vi "RT_P3.vi"() -> ()   [LabVIEW 2014]
uses:
  <vilib>/Utility/RT CPU Load.ctl
  <vilib>/Platform/TimedLoop/XDataNode/timing_clust.ctl
  <vilib>/Platform/TimedLoop/XDataNode/nitl_modes.ctl
  <vilib>/Platform/TimedLoop/XDataNode/wakeup.ctl
  <vilib>/RioEmbeddedCAN/RioEmbeddedCAN.llb/CANFilterMode.ctl
  <vilib>/RioEmbeddedCAN/RioEmbeddedCAN.llb/CANFilterSetting.ctl
  <vilib>/FPGAPlugInAG/sbRIO-9636/niLvFpga_Open_sbRIO-9636.vi
  <vilib>/FPGAPlugInAG/sbRIO-9636/niLvFpga_Close_sbRIO-9636.vi
  <vilib>/Instr/_visa.llb/VISA Configure Serial Port (Instr).vi
  <vilib>/rvi/interface/common/dynamic/niFpgaDynamicAddResources.vi
  <vilib>/FPGAPlugInAG/Dynamic/niLvFpga_Reset_Dynamic.vi
  <vilib>/FPGAPlugInAG/Dynamic/niLvFpga_Run_Dynamic.vi
  <vilib>/Utility/error.llb/Error Cluster From Error Code.vi
  <vilib>/rvi/errors/niLvFpgaAdjustHostInterfaceError.vi
  <vilib>/FPGAPlugInAG/Dynamic/niLvFpga_Close_Dynamic.vi
  <vilib>/Platform/TimedLoop/XDataNode/XDataNode.xnode
  Z:/cloud/LabView/roger-i2c/Host API/Controls/FPGA I2C_FPGA Ref.ctl
  <vilib>/rvi/interface/nirviOpenFPGA/nirviOpenFPGA.xnode
  FPGA bitfiles/telemetriap3_FPGATarget_fpgaprova_w0avayymtNg.lvbitx
  fpga_p3.vi
  <vilib>/rvi/interface/nirviCloseFPGA/nirviCloseFPGA.xnode
  <vilib>/rvi/interface/nirviMethod/nirviMethod.xnode
  <vilib>/rvi/interface/nirviReadWriteControl/nirviReadWriteControl.xnode
  <vilib>/Platform/TimedLoop/XDataNode/XDNodeRunTimeDep.lvlib
  <vilib>/NI_Real-Time Target Support.lvlib
  <vilib>/FPGAPlugInAG/Dynamic/niLvFpga_ReadFifo_Dynamic.vi
  <vilib>/rvi/errors/niLvFpgaMergeErrorWithErrorCode.vi
  <vilib>/FPGAPlugInAG/Dynamic/niLvFpga_StartFifo_Dynamic.vi
  NiFpgaLv.dll
  <vilib>/rvi/interface/Simulation/niFpgaSimulationCallBeginRW.vi
panel:
  out "a-z":dbl
  out "a-y":dbl
  out "a-x":dbl
  out "CPU loads":T1[](array[typedef]) {"ISR (%)" format="%#.2f"; "Idle (%)" format="%#.2f"; "Background (%)" format="%#.2f"; "Normal (%)" format="%#.2f"; "Above Normal (%)" format="%#.2f"; "High (%)" format="%#.2g"; "Timed Structures (%)" format="%#.2g"; "Time Critical (%)" format="%#.2g"; "Total (%)" format="%#.2g"}
  out "g-z":dbl
  out "g-y":dbl
  out "g-x":dbl
  out "Error rs-232 display":errorcluster
  in  "Buzzer":bool
  in  "STOP LIGHT":bool
  out "Brake Sensor \nFront":sgl
  out "error out save file":errorcluster
  out "Brake Sensor \nRear":sgl
  out "Steering anlge":sgl
  out "overflow?":bool
  in  "stop":bool
  out "=< 10?":bool
  out "Loop Time":u32
  out "Fifo Overflow?":bool
  out "Elements Remaining after":u32
  out "F-L":sgl
  out "R-R":sgl
  out "F-R":sgl
  out "R-L":sgl
  out "Elements Remaining before":u32
  out "error out fpga":errorcluster
  out "Drive Speed":sgl
  out "Fuel Used":sgl
  out "Gear":u16
  out "Oil Temp":sgl
  out "Oil Pressure":sgl
  out "Battery Voltage":sgl
  out "Engine Temp":sgl
  out "Throttle":sgl
  out "Lambda":sgl
  out "Air Temp":sgl
  out "Map (bar)":sgl
  out "Rpm":u16
  out "error out can":errorcluster
  # "CAN MOTEC"
  # "FPGA"
  # "Telemetria delle telemetria"
  # "I2C\nI2C\nI2C Sistema inerziale"
  # "Indirizzo 2"
  # "Indirizzo 3"
  # "Indirizzo 4"
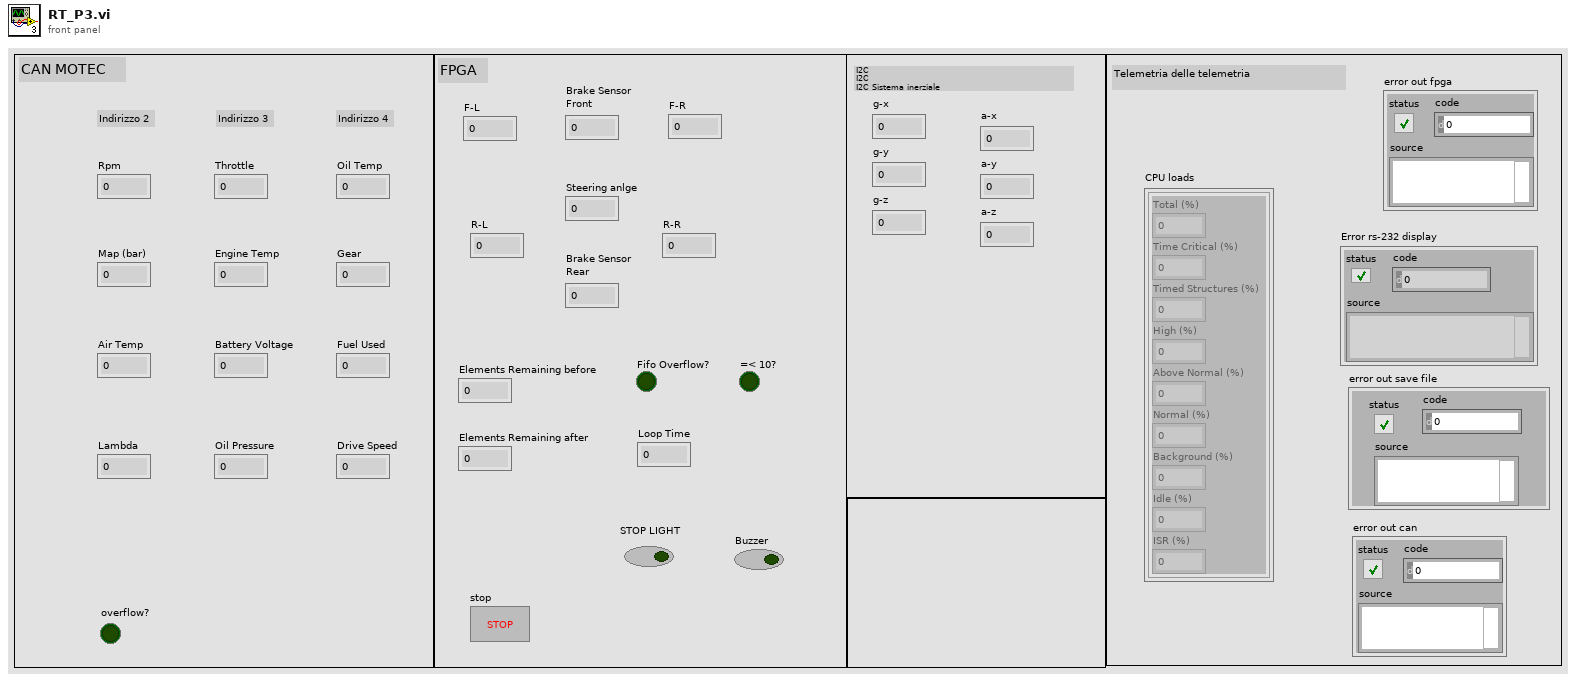
[diagram p1: front panel]
types:
  T1 = typedef "NI_Real-Time Target Support.lvlib/RT CPU Load.ctl" = cluster{"Total (%)":dbl, "Time Critical (%)":dbl, "Timed Structures (%)":dbl, "High (%)":dbl, "Above Normal (%)":dbl, "Normal (%)":dbl, "Background (%)":dbl, "Idle (%)":dbl, "ISR (%)":dbl}
  T2 = typedef "XDNodeRunTimeDep.lvlib/timing_clust.ctl" = cluster{"Expected End [f-1]":u64, "Actual End [f-1]":u64, "Finished Late? [f-1]":bool, "Expected End [i-1]":u64, "Actual End [i-1]":u64, "Finished Late? [i-1]":bool, "Expected Start [i]":u64, "Actual Start [i]":u64, "Expected Start [f]":u64, "Actual Start [f]":u64, "Source Name":string, "Structure Name":string, "Period":i64, "Deadline":i64, "Offset":i64, "Start":i64, "Priority":i32, "Timeout":i32, "Mode":T3, "Wakeup Reason":T4, "Error":errorcluster, "Source Type":string, "Secondary Source Type":string, "Global End Time":u64, "Global Start Time":u64, "Frame Duration":u64, "Iteration Duration":u64, "Assigned CPU":i32, "I/O Scan Engine Mode":u32}
  T3 = typedef "XDNodeRunTimeDep.lvlib/nitl_modes.ctl" = enum32{"No Change", "Process missed periods, maintain original phase", "Discard missed periods, maintain original phase", "Process missed periods, ignore original phase", "Discard missed periods, ignore original phase"}
  T4 = typedef "XDNodeRunTimeDep.lvlib/wakeup.ctl" = enum32{"Normal", "Aborted", "Asynchronous wakeup", "Timing source error", "Timed loop error", "Timeout"}
  T5 = typedef "CANFilterSetting.ctl" = cluster{"identifier":u32, "identifier mask":u32, "extended?":bool, "RTR?":bool, "RTR mask?":bool}
  T6 = typedef "CANFilterMode.ctl" = enum16{"Disabled", "32-bit", "16-bit", "8-bit"}
  T7 = typedef "CANFrameControl.ctl" = cluster{"identifier":u32, "extended?":bool, "type":u8, "payload":u8[]}
  T8 = enum16{"open", "open or create", "create or replace", "create", "open (read-only)"}
  T9 = typedef "FPGA I2C_FPGA Ref.ctl" = refnum<k20>
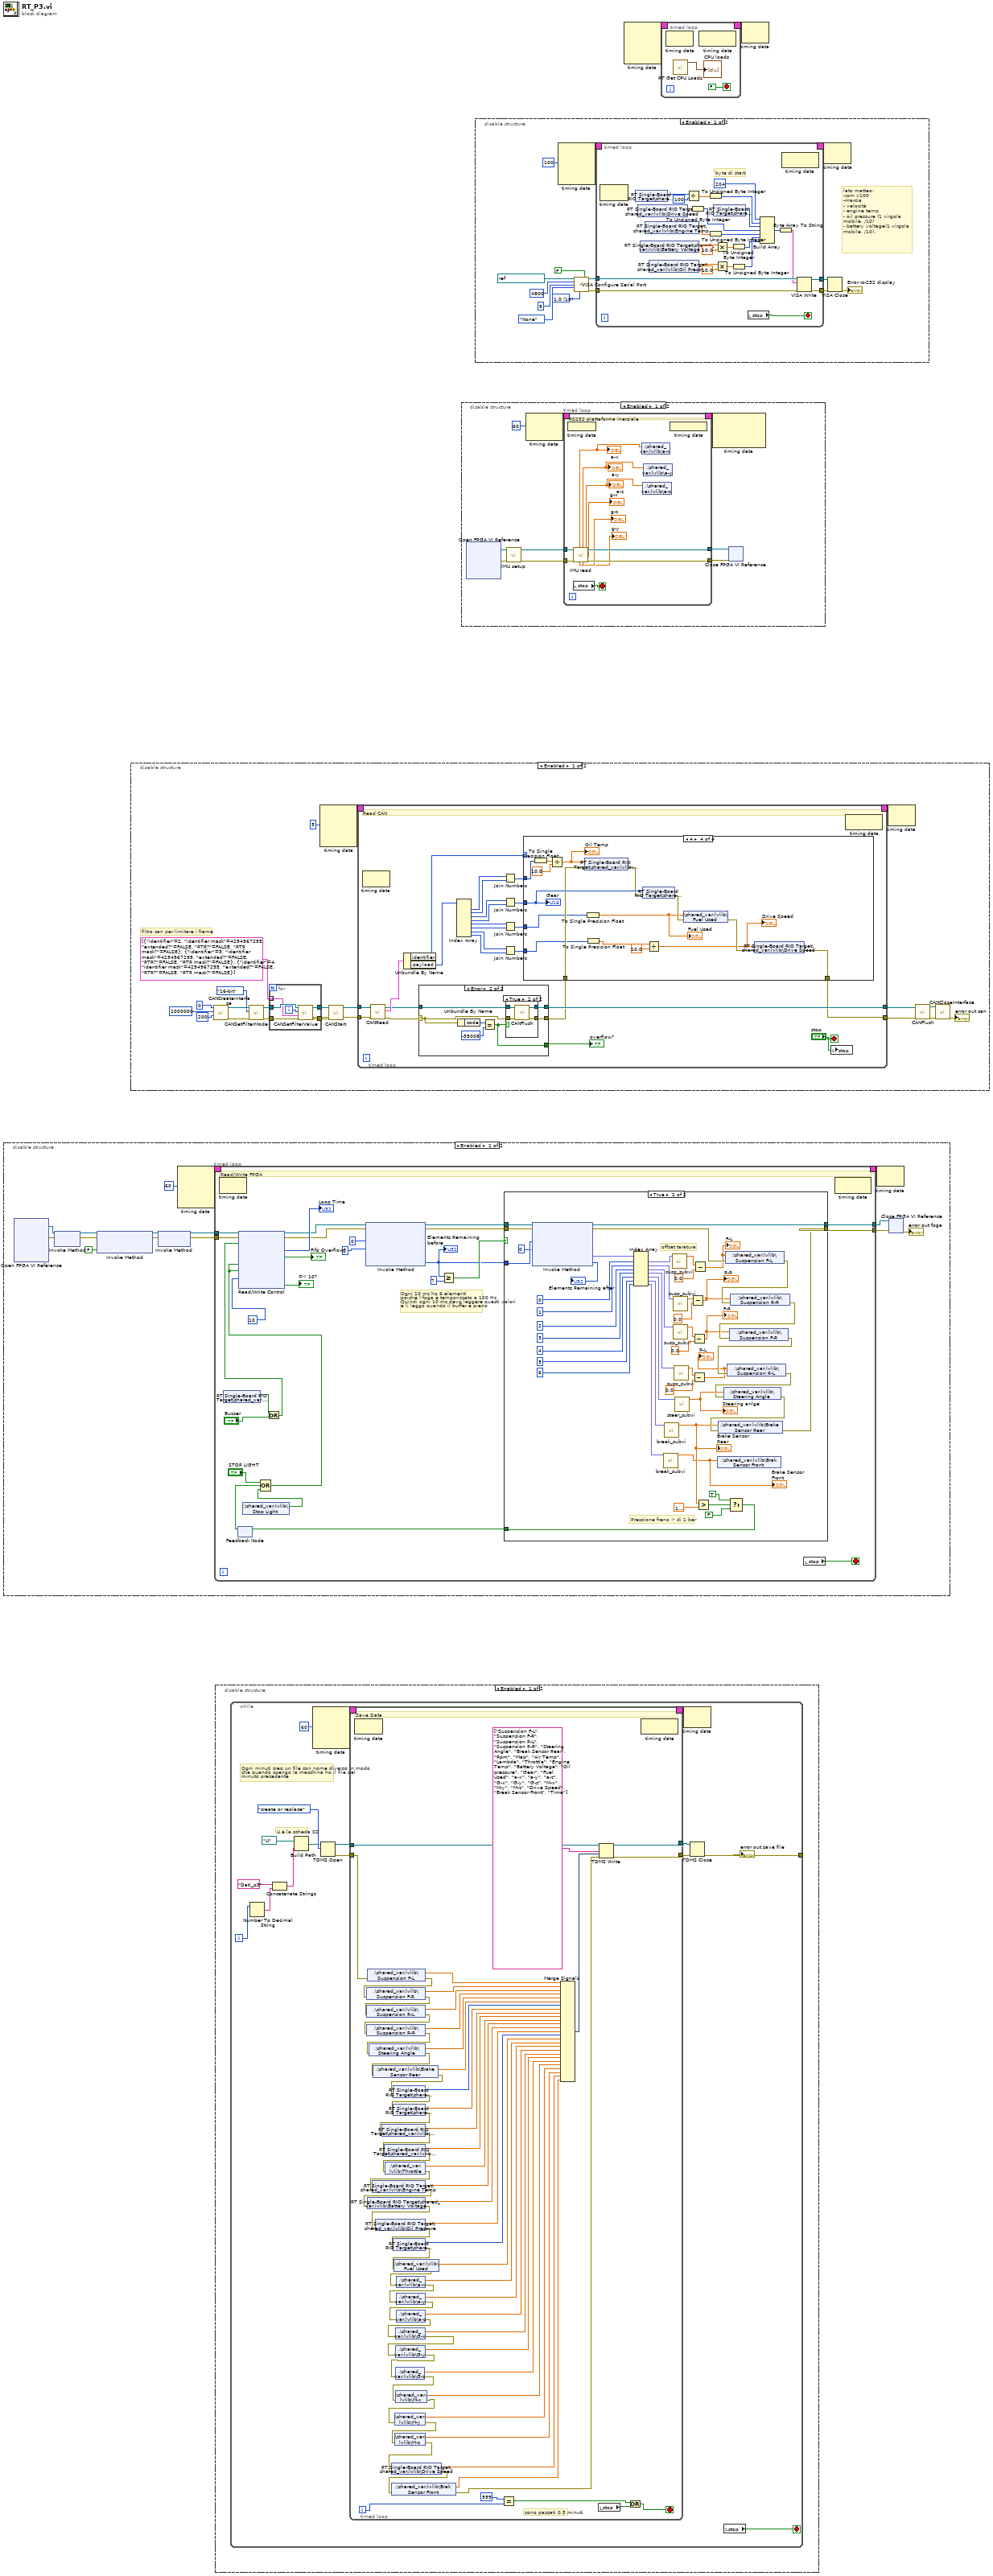
[diagram p0: block diagram]
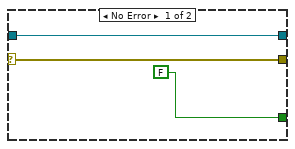
[diagram p4: hidden frame]
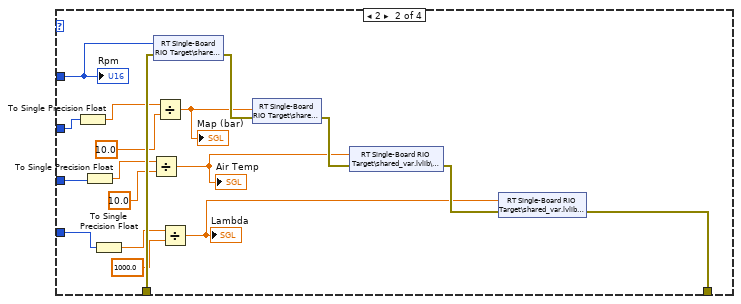
[diagram p7: hidden frame]
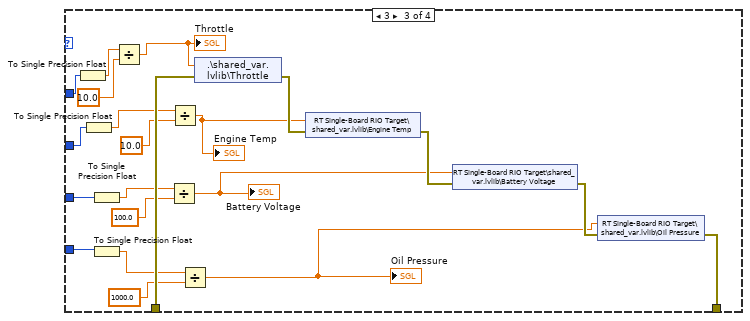
[diagram p8: hidden frame]
diagram:
  n1 = disable-structure shown="Enabled" {
    frame Enabled {
      n2 = xnode "Open FPGA VI Reference"() -> ("FPGA VI Reference Out"=w15:refnum<k20>, "error out"=w14:errorcluster)  [unwired: 2 in]
      n3 = xnode "Invoke Method"("FPGA VI Reference In"=w15, "error in"=w14) -> ("FPGA VI Reference Out"=w12:refnum<k20>, "error out"=w11:errorcluster)
      n4 = xnode "Invoke Method"("FPGA VI Reference In"=w12, "error in"=w11, "Wait Until Done (F)"=FALSE) -> ("FPGA VI Reference Out"=w7:refnum<k20>, "error out"=w6:errorcluster)
      n5 = xnode "Invoke Method"("FPGA VI Reference In"=w7, "error in"=w6) -> ("FPGA VI Reference Out"=w5:refnum<k20>, "error out"=w4:errorcluster)
      n6 = node-c288(i64 60 ("Period")) -> (w17:T2)  [unwired: 3 in]
      n7 = timed-loop {
        tunnel: [w33] -> w9
        tunnel: [w32] -> w8
        tunnel: w5 -> [w31]
        tunnel: w4 -> [w30]
        timing: w17 -> [_]
        timing-out: [_] -> w16
        stop <- w27 stop-if-true
        # "Ogni 10 ms ho 6 elementi\npoichè l'fpga è temporizzato a 100 Hz\nQuindi ogni 10 ms devo leggere questi valori\ne li leggo quando il buffer è pieno"
        # "Read/Write FPGA"
        n8 = node-c288() -> ()  [unwired: 1 in, 1 out]
        n9 = shared-variable "RT Single-Board RIO Target\\shared_var.lvlib\\Buzzer"() -> (w23:bool)  [unwired: 1 in, 1 out]
        n10 = feedback #1() -> (w19:bool)  [unwired: 1 in]
        n11 = shared-variable ".\\shared_var.lvlib\\Stop Light"() -> (w18:bool)  [unwired: 1 in, 1 out]
        n12 = Compound Arithmetic op=OR("STOP LIGHT", w19, w18) -> (w21:bool)
        n13 = Or(x=w23, y="Buzzer") -> (x .or. y?=w22:bool)
        n14 = xnode "Read/Write Control"("FPGA VI Reference In"=w31, "error in"=w30, "Buzzer"=w22, "FPGA LED"=w21, "Stop Light"=w21, "Count(uSec)"=u32 10 ("Count(mSec)")) -> ("FPGA VI Reference Out"=w29:refnum<k20>, "error out"=w34:errorcluster, "Loop Time"=→"Loop Time":u32, "Fifo Overflow?"=→"Fifo Overflow?":bool, "=< Lopp time?"=→"=< 10?":bool)
        n15 = xnode "Invoke Method"("FPGA VI Reference In"=w29, "error in"=w34, "Number of Elements"=u32 0, "Timeout (ms)"=0) -> ("FPGA VI Reference Out"=w40:refnum<k20>, "error out"=w39:errorcluster, "Elements Remaining"=w35:u32)  [unwired: 1 out]
        "Elements Remaining before" <- w35
        n16 = Greater Or Equal?(x=w35, y=u32 7) -> (x >= y?=w37:bool)
        n17 = case shown="True" w37 {
          tunnel: w40 -> [w47 w95]
          tunnel: w39 -> [w46 w94]
          tunnel: [w47 w93] -> w33
          tunnel: [w46 w83] -> w32
          tunnel: w35 -> [_ w92]
          tunnel: [_ w88] -> w28
          frame False {
          }
          frame True {
            # "offset taratura"
            # "Pressione freno > di 1 bar"
            n18 = xnode "Invoke Method"("FPGA VI Reference In"=w95, "error in"=w94, "Number of Elements"=w92, "Timeout (ms)"=0) -> ("FPGA VI Reference Out"=w93:refnum<k20>, "error out"=w85:errorcluster, "Data"=w82:fxp<+,32,3>[], "Elements Remaining"=→"Elements Remaining after":u32)
            n19 = Index Array(array=w82, index #1=0 ("index"), index #2=1 ("index"), index #3=2 ("index"), index #4=3 ("index"), index #5=4 ("index"), index #6=5 ("index"), index #7=6 ("index")) -> (element #1=w73:fxp<+,32,3>, element #2=w72:fxp<+,32,3>, element #3=w71:fxp<+,32,3>, element #4=w70:fxp<+,32,3>, element #5=w69:fxp<+,32,3>, element #6=w67:fxp<+,32,3>, element #7=w49:fxp<+,32,3>)
            n20 = call "break_subvi.vi"("Numeric in"=w49) -> ("Numeric out"=w48:sgl)  [unwired: 10 in]
            "Brake Sensor \nFront" <- w48
            n21 = call "break_subvi.vi"("Numeric in"=w67) -> ("Numeric out"=w50:sgl)  [unwired: 10 in]
            "Brake Sensor \nRear" <- w50
            n22 = call "susp_subvi.vi"("Numeric in"=w73) -> ("Numeric out"=w62:sgl)  [unwired: 10 in]
            n23 = call "susp_subvi.vi"("Numeric in"=w72) -> ("Numeric out"=w55:sgl)  [unwired: 10 in]
            n24 = call "susp_subvi.vi"("Numeric in"=w71) -> ("Numeric out"=w59:sgl)  [unwired: 10 in]
            n25 = call "susp_subvi.vi"("Numeric in"=w70) -> ("Numeric out"=w53:sgl)  [unwired: 10 in]
            n26 = call "steer_subvi.vi"("Numeric in"=w69) -> ("Numeric out"=w68:sgl)  [unwired: 10 in]
            "Steering anlge" <- w68
            n27 = Subtract(x=w55, y=sgl 0.0 ("Off R-R")) -> (x-y=w56:sgl)
            "R-R" <- w56
            n28 = Subtract(x=w59, y=sgl 0.0 ("Off F-R")) -> (x-y=w58:sgl)
            "F-R" <- w58
            n29 = Subtract(x=w53, y=sgl 0.0 ("Off R-L")) -> (x-y=w52:sgl)
            "R-L" <- w52
            n30 = Subtract(x=w62, y=sgl 0.0 ("Off F-L")) -> (x-y=w61:sgl)
            "F-L" <- w61
            n31 = Greater?(x=w50, y=sgl 1.7) -> (0:w89:bool)
            n32 = shared-variable ".\\shared_var.lvlib\\Brak Sensor Front"(w48) -> ()  [unwired: 1 in, 1 out]
            n33 = shared-variable ".\\shared_var.lvlib\\Suspension F-L"(w61, error in=w85) -> (error out=w66:errorcluster)
            n34 = Select(t=TRUE, s=w89, f=FALSE) -> (s? t:f=w88:bool)
            n35 = shared-variable ".\\shared_var.lvlib\\Suspension R-R"(w56, error in=w66) -> (error out=w65:errorcluster)
            n36 = shared-variable ".\\shared_var.lvlib\\Suspension F-R"(w58, error in=w65) -> (error out=w63:errorcluster)
            n37 = shared-variable ".\\shared_var.lvlib\\Suspension R-L"(w52, error in=w63) -> (error out=w64:errorcluster)
            n38 = shared-variable ".\\shared_var.lvlib\\Steering Angle"(w68, error in=w64) -> (error out=w84:errorcluster)
            n39 = shared-variable ".\\shared_var.lvlib\\Brake Sensor Rear"(w50, error in=w84) -> (error out=w83:errorcluster)
          }
        }
        n40 = feedback-in #1(w28) -> ()
        n41 = local read "stop"() -> (w27:bool)
        n42 = node-c288() -> ()  [unwired: 1 in, 1 out]
      }
      n43 = node-c288(w16) -> ()  [unwired: 1 out]
      n44 = xnode "Close FPGA VI Reference"("FPGA VI Reference In"=w9, "error in"=w8) -> ("error out"=→"error out fpga":errorcluster)
    }
    frame Disabled {
    }
  }
  n45 = disable-structure shown="Enabled" {
    frame Enabled {
      # "filtro can per limitare i frame"
      n46 = call <vilib>:"CANCreateInterface.vi"("receive queue size (5)"=u32 200, "baud rate (125000 bps)"=u32 1000000, "interface index"=u32 0) -> ("error out"=w115:errorcluster, "interface object out"=w116:refnum<k20>)  [unwired: 7 in]
      n47 = call <vilib>:"CANSetFilterMode.vi"("error in (no error)"=w115, "filter mode (32-bit)"=CANFilterMode."16-bit", "interface object in"=w116) -> ("error out"=w117:errorcluster, "interface object out"=w118:refnum<k20>)  [unwired: 7 in]
      n48 = for {
        tunnel: T5[] [{"identifier"=2, "identifier mask"=4294967295, "extended?"=FALSE, "RTR?"=FALSE, "RTR mask?"=FALSE}, {"identifier"=3, "identifier mask"=4294967295, "extended?"=FALSE, "RTR?"=FALSE, "RTR mask?"=FALSE}, {"identifier"=4, "identifier mask"=4294967295, "extended?"=FALSE, "RTR?"=FALSE, "RTR mask?"=FALSE}] ("Array") -> [w225] mode=indexing
        tunnel: w118 -> [w228]
        tunnel: [w227] -> w113
        tunnel: w117 -> [w223]
        tunnel: [w226] -> w112
        i -> [w224]
        n49 = call <vilib>:"CANSetFilterValue.vi"("error in (no error)"=w223, "filter frame"=w225, "filter index (0)"=w224, "interface object in"=w228) -> ("error out"=w226:errorcluster, "interface object out"=w227:refnum<k20>)  [unwired: 6 in]
      }
      n50 = node-c288(i64 5 ("Period")) -> (w120:T2)  [unwired: 3 in]
      n51 = call <vilib>:"CANStart.vi"("error in (no error)"=w112, "interface object in"=w113) -> ("error out"=w110:errorcluster, "interface object out"=w111:refnum<k20>)  [unwired: 8 in]
      n52 = timed-loop {
        tunnel: w111 -> [w143]
        tunnel: w110 -> [w144]
        tunnel: [w126] -> w104
        timing: w120 -> [_]
        timing-out: [_] -> w119
        tunnel: [w127] -> w102
        stop <- "stop" stop-if-true
        # "Read CAN"
        n53 = node-c288() -> ()  [unwired: 1 in, 1 out]
        n54 = call <vilib>:"CANRead.vi"("error in (no error)"=w144, "interface object in"=w143) -> ("error out"=w125:errorcluster, "CAN frame"=w142:T7, "interface object out"=w121:refnum<k20>)  [unwired: 6 in, 1 out]
        n55 = Unbundle By Name(w142) -> ("identifier"=w132:u32, "payload"=w133:u8[])
        n56 = case shown="Error" w125 {
          selector: w125 -> [w147 w150]
          tunnel: [w147 w151] -> w124
          tunnel: w121 -> [w146 w148]
          tunnel: [w146 w152] -> w127
          tunnel: [FALSE w149] -> w122
          frame No Error {
          }
          frame Error {
            n57 = Unbundle By Name(w150) -> ("code"=w154:i32)
            n58 = Equal?(x=w154, y=-35008) -> (x = y?=w149:bool)
            n59 = case shown="True" w149 {
              tunnel: w150 -> [w156 w158]
              tunnel: w148 -> [w155 w160]
              tunnel: [w155 w159] -> w152
              tunnel: [w156 w157] -> w151
              frame False {
              }
              frame True {
                n60 = call <vilib>:"CANFlush.vi"("error in (no error)"=w158, "interface object in"=w160) -> ("error out"=w157:errorcluster, "interface object out"=w159:refnum<k20>)  [unwired: 8 in]
              }
            }
          }
        }
        "overflow?" <- w122
        n61 = Index Array(array=w133) -> (element #1=w141:u8, element #2=w140:u8, element #3=w139:u8, element #4=w138:u8, element #5=w137:u8, element #6=w136:u8, element #7=w135:u8, element #8=w134:u8)  [unwired: 8 in]
        n62 = Join Numbers(hi=w141, lo=w140) -> ((hi.lo)=w131:u16)
        n63 = Join Numbers(hi=w139, lo=w138) -> ((hi.lo)=w130:u16)
        n64 = Join Numbers(hi=w137, lo=w136) -> ((hi.lo)=w129:u16)
        n65 = Join Numbers(hi=w135, lo=w134) -> ((hi.lo)=w128:u16)
        n66 = case shown="4" w132 {
          tunnel: w131 -> [_ w181 w196 w213]
          tunnel: w130 -> [_ w166 w190 w218]
          tunnel: w129 -> [_ w175 w195 w209]
          tunnel: w128 -> [_ w173 w185 w210]
          tunnel: w124 -> [w163 w180 w202 w217]
          tunnel: [w163 w176 w198 w207] -> w126
          frame 0, Default {
          }
          frame 2 {
            n67 = To Single Precision Float(number=w166) -> (single precision float=w165:sgl)
            n68 = To Single Precision Float(number=w175) -> (single precision float=w168:sgl)
            n69 = To Single Precision Float(number=w173) -> (single precision float=w170:sgl)
            n70 = Divide(x=w168, y=sgl 10.0 ("x")) -> (x/y=w174:sgl)
            "Air Temp" <- w174
            n71 = shared-variable "RT Single-Board RIO Target\\shared_var.lvlib\\Rpm"(w181, error in=w180) -> (error out=w179:errorcluster)
            n72 = Divide(x=w165, y=sgl 10.0 ("x")) -> (x/y=w164:sgl)
            "Map (bar)" <- w164
            n73 = Divide(x=w170, y=sgl 1000.0 ("x")) -> (x/y=w172:sgl)
            "Lambda" <- w172
            n74 = shared-variable "RT Single-Board RIO Target\\shared_var.lvlib\\Map"(w164, error in=w179) -> (error out=w178:errorcluster)
            n75 = shared-variable "RT Single-Board RIO Target\\shared_var.lvlib\\Air Temp"(w174, error in=w178) -> (error out=w177:errorcluster)
            n76 = shared-variable "RT Single-Board RIO Target\\shared_var.lvlib\\Lambda"(w172, error in=w177) -> (error out=w176:errorcluster)
            "Rpm" <- w181
          }
          frame 3 {
            n77 = To Single Precision Float(number=w196) -> (single precision float=w192:sgl)
            n78 = To Single Precision Float(number=w190) -> (single precision float=w187:sgl)
            n79 = To Single Precision Float(number=w195) -> (single precision float=w191:sgl)
            n80 = To Single Precision Float(number=w185) -> (single precision float=w184:sgl)
            n81 = Divide(x=w192, y=sgl 10.0 ("x")) -> (x/y=w197:sgl)
            "Throttle" <- w197
            n82 = Divide(x=w191, y=sgl 100.0) -> (x/y=w194:sgl)
            "Battery Voltage" <- w194
            n83 = Divide(x=w187, y=sgl 10.0 ("x")) -> (x/y=w189:sgl)
            "Engine Temp" <- w189
            n84 = Divide(x=w184, y=1000.0 ("x")) -> (x/y=w183:dbl)
            "Oil Pressure" <- w183
            n85 = shared-variable ".\\shared_var.lvlib\\Throttle"(w197, error in=w202) -> (error out=w201:errorcluster)
            n86 = shared-variable "RT Single-Board RIO Target\\shared_var.lvlib\\Engine Temp"(w189, error in=w201) -> (error out=w200:errorcluster)
            n87 = shared-variable "RT Single-Board RIO Target\\shared_var.lvlib\\Battery Voltage"(w194, error in=w200) -> (error out=w199:errorcluster)
            n88 = shared-variable "RT Single-Board RIO Target\\shared_var.lvlib\\Oil Pressure"(w183, error in=w199) -> (error out=w198:errorcluster)
          }
          frame 4 {
            n89 = To Single Precision Float(number=w213) -> (single precision float=w212:sgl)
            n90 = Divide(x=w212, y=sgl 10.0) -> (x/y=w214:sgl)
            "Oil Temp" <- w214
            n91 = shared-variable "RT Single-Board RIO Target\\shared_var.lvlib\\Oil Temp"(w214, error in=w217) -> (error out=w216:errorcluster)
            n92 = To Single Precision Float(number=w209) -> (single precision float=w206:sgl)
            "Fuel Used" <- w206
            n93 = To Single Precision Float(number=w210) -> (single precision float=w205:sgl)
            n94 = shared-variable "RT Single-Board RIO Target\\shared_var.lvlib\\Gear"(w218, error in=w216) -> (error out=w215:errorcluster)
            n95 = Divide(x=w205, y=sgl 10.0) -> (x/y=w204:sgl)
            "Drive Speed" <- w204
            n96 = shared-variable ".\\shared_var.lvlib\\Fuel Used"(w206, error in=w215) -> (error out=w208:errorcluster)
            n97 = shared-variable "RT Single-Board RIO Target\\shared_var.lvlib\\Drive Speed"(w204, error in=w208) -> (error out=w207:errorcluster)
            "Gear" <- w218
          }
        }
        n98 = local write "stop"("stop") -> ()
        n99 = node-c288() -> ()  [unwired: 1 in, 1 out]
      }
      n100 = node-c288(w119) -> ()  [unwired: 1 out]
      n101 = call <vilib>:"CANFlush.vi"("error in (no error)"=w104, "interface object in"=w102) -> ("error out"=w103:errorcluster, "interface object out"=w105:refnum<k20>)  [unwired: 8 in]
      n102 = call <vilib>:"CANCloseInterface.vi"("error in (no error)"=w103, "interface object in"=w105) -> ("error out"=→"error out can":errorcluster)  [unwired: 9 in]
    }
    frame Disabled {
    }
  }
  n103 = disable-structure shown="Enabled" {
    frame Enabled {
      n104 = while {
        tunnel: [w235] -> w229
        i -> [w234]
        stop <- w241 stop-if-true
        # "Ogni minuti creo un file con nome diverso in modo\nche quando spengo la macchina ho il file del \nminuto precedente"
        # "U è la scheda SD"
        n105 = Number To Decimal String(number=w234) -> (decimal integer string=w238:string)  [unwired: 1 in]
        n106 = Concatenate Strings("Dati_p3" ("name or relative path"), w238) -> (w239:string)
        n107 = Build Path(base path=path "U:/", name or relative path=w239) -> (appended path=w233:path)
        n108 = node-c288(i64 60 ("Period")) -> (w232:T2)  [unwired: 3 in]
        n109 = TDMS Open(10:T8."create or replace" ("operation (0:open)"), 11:w233) -> (0:w237:errorcluster, 3:w244:refnum<k34>)  [unwired: 5 in]
        n110 = timed-loop {
          tunnel: w244 -> [w261]
          tunnel: [w247] -> w242
          tunnel: w237 -> [w287]
          tunnel: [w246] -> w236
          timing: w232 -> [_]
          timing-out: [_] -> w231
          i -> [w303]
          stop <- w310 stop-if-true
          # "sono passati 0.5 minuti"
          # "Save Data"
          n111 = node-c288() -> ()  [unwired: 1 in, 1 out]
          n112 = shared-variable ".\\shared_var.lvlib\\Suspension F-L"(error in=w287) -> (w306:sgl, error out=w286:errorcluster)
          n113 = shared-variable ".\\shared_var.lvlib\\Suspension F-R"(error in=w286) -> (w305:sgl, error out=w285:errorcluster)
          n114 = shared-variable ".\\shared_var.lvlib\\Suspension R-L"(error in=w285) -> (w298:sgl, error out=w284:errorcluster)
          n115 = shared-variable ".\\shared_var.lvlib\\Suspension R-R"(error in=w284) -> (w304:sgl, error out=w283:errorcluster)
          n116 = shared-variable ".\\shared_var.lvlib\\Steering Angle"(error in=w283) -> (w300:sgl, error out=w282:errorcluster)
          n117 = shared-variable ".\\shared_var.lvlib\\Brake Sensor Rear"(error in=w282) -> (w299:sgl, error out=w281:errorcluster)
          n118 = shared-variable "RT Single-Board RIO Target\\shared_var.lvlib\\Rpm"(error in=w281) -> (w297:u16, error out=w280:errorcluster)
          n119 = shared-variable "RT Single-Board RIO Target\\shared_var.lvlib\\Map"(error in=w280) -> (w296:sgl, error out=w279:errorcluster)
          n120 = shared-variable "RT Single-Board RIO Target\\shared_var.lvlib\\Air Temp"(error in=w279) -> (w295:sgl, error out=w278:errorcluster)
          n121 = shared-variable "RT Single-Board RIO Target\\shared_var.lvlib\\Lambda"(error in=w278) -> (w294:sgl, error out=w277:errorcluster)
          n122 = shared-variable ".\\shared_var.lvlib\\Throttle"(error in=w277) -> (w293:sgl, error out=w276:errorcluster)
          n123 = shared-variable "RT Single-Board RIO Target\\shared_var.lvlib\\Engine Temp"(error in=w276) -> (w292:sgl, error out=w275:errorcluster)
          n124 = shared-variable "RT Single-Board RIO Target\\shared_var.lvlib\\Battery Voltage"(error in=w275) -> (w291:sgl, error out=w274:errorcluster)
          n125 = shared-variable "RT Single-Board RIO Target\\shared_var.lvlib\\Oil Pressure"(error in=w274) -> (w290:sgl, error out=w273:errorcluster)
          n126 = shared-variable "RT Single-Board RIO Target\\shared_var.lvlib\\Gear"(error in=w273) -> (w289:u8, error out=w272:errorcluster)
          n127 = shared-variable ".\\shared_var.lvlib\\Fuel Used"(error in=w272) -> (w288:sgl, error out=w271:errorcluster)
          n128 = shared-variable ".\\shared_var.lvlib\\a-x"(error in=w271) -> (w266:dbl, error out=w270:errorcluster)
          n129 = shared-variable ".\\shared_var.lvlib\\a-y"(error in=w270) -> (w265:dbl, error out=w269:errorcluster)
          n130 = shared-variable ".\\shared_var.lvlib\\a-z"(error in=w269) -> (w264:dbl, error out=w268:errorcluster)
          n131 = shared-variable ".\\shared_var.lvlib\\G-x"(error in=w268) -> (w262:dbl, error out=w267:errorcluster)
          n132 = shared-variable ".\\shared_var.lvlib\\G-y"(error in=w267) -> (w263:dbl, error out=w260:errorcluster)
          n133 = shared-variable ".\\shared_var.lvlib\\G-z"(error in=w260) -> (w255:dbl, error out=w259:errorcluster)
          n134 = shared-variable ".\\shared_var.lvlib\\M-x"(error in=w259) -> (w254:dbl, error out=w258:errorcluster)
          n135 = shared-variable ".\\shared_var.lvlib\\M-y"(error in=w258) -> (w253:dbl, error out=w257:errorcluster)
          n136 = shared-variable ".\\shared_var.lvlib\\M-z"(error in=w257) -> (w252:dbl, error out=w256:errorcluster)
          n137 = shared-variable "RT Single-Board RIO Target\\shared_var.lvlib\\Drive Speed"(error in=w256) -> (w251:dbl, error out=w250:errorcluster)
          n138 = shared-variable ".\\shared_var.lvlib\\Brak Sensor Front"(error in=w250) -> (w248:sgl, error out=w249:errorcluster)
          n139 = Equal?(x=999, y=w303) -> (x = y?=w301:bool)
          n140 = Merge Signals(w306, w305, w298, w304, w300, w299, w297, w296, w295, w294, w293, w292, w291, w290, w289, w288, w266, w265, w264, w262, w263, w255, w254, w253, w252, w251, w248) -> (w307:dynamicdata)
          n141 = local read "stop"() -> (w309:bool)
          n142 = TDMS Write(0:w261, 7:string[] ["Suspension F-L", "Suspension F-R", "Suspension R-L", "Suspension R-R", "Steering Angle", "Break Sensor Rear", "Rpm", "Map", "Air Temp", "Lambda", "Throttle", "Engine Temp", "Battery Voltage", "Oil pressure", "Gear", "Fuel Used", "a-x", "a-y", "a-z", "G-x", "G-y", "G-z", "M-x", "M-y", "M-z", "Drive Speed", "Break Sensor Front", "Time"] ("channel name(s) in (Untitled)"), 9:w307, 11:w249) -> (4:w247:refnum<k34>, 15:w246:errorcluster)  [unwired: 2 in, 2 out]
          n143 = Or(x=w301, y=w309) -> (x .or. y?=w310:bool)
          n144 = node-c288() -> ()  [unwired: 1 in, 1 out]
        }
        n145 = node-c288(w231) -> ()  [unwired: 1 out]
        n146 = TDMS Close(8:w236, 11:w242) -> (0:w235:errorcluster)  [unwired: 1 out]
        n147 = local read "stop"() -> (w241:bool)
      }
      "error out save file" <- w229
    }
    frame Disabled {
    }
  }
  n148 = disable-structure shown="Enabled" {
    frame Enabled {
      n149 = xnode "Open FPGA VI Reference"() -> ("FPGA VI Reference Out"=w323:T9, "error out"=w322:errorcluster)  [unwired: 2 in]
      n150 = call "IMU setup.vi"("error in (no error)"=w322, "Refnum in"=w323) -> ("error out"=w320:errorcluster, "Refnum out"=w321:T9)  [unwired: 8 in]
      n151 = node-c288(i64 60 ("Period")) -> (w325:T2)  [unwired: 1 in]
      n152 = timed-loop {
        timing: w325 -> [_]
        timing-out: [_] -> w324
        tunnel: w320 -> [w335]
        tunnel: w321 -> [w334]
        tunnel: [w333] -> w318
        tunnel: [w332] -> w319
        stop <- w336 stop-if-true
        # "RS232 piattaforma inerziale"
        n153 = node-c288() -> ()  [unwired: 1 in]
        n154 = local read "stop"() -> (w336:bool)
        n155 = call "IMU read.vi"("error in (no error)"=w335, "Refnum in"=w334) -> ("error out"=w333:errorcluster, "g-x"=→"g-x":dbl, "a-z"=w327:dbl, "Refnum out"=w332:T9, "g-z"=→"g-z":dbl, "a-y"=w326:dbl, "g-y"=→"g-y":dbl, "a-x"=w328:dbl)  [unwired: 2 in]
        "a-x" <- w328
        "a-y" <- w326
        "a-z" <- w327
        n156 = shared-variable ".\\shared_var.lvlib\\a-x"(w328) -> ()  [unwired: 1 in, 1 out]
        n157 = shared-variable ".\\shared_var.lvlib\\a-z"(w327) -> ()  [unwired: 1 in, 1 out]
        n158 = shared-variable ".\\shared_var.lvlib\\a-y"(w326) -> ()  [unwired: 1 in, 1 out]
        n159 = node-c288() -> ()  [unwired: 1 out]
      }
      n160 = node-c288(w324) -> ()  [unwired: 3 out]
      n161 = xnode "Close FPGA VI Reference"("FPGA VI Reference In"=w319, "error in"=w318) -> ()  [unwired: 1 out]
    }
    frame Disabled {
    }
  }
  n162 = disable-structure shown="Enabled" {
    frame Enabled {
      w344 = u16 10 items=["1.0"=10, "1.5"=15, "2.0"=20] ("stop bits (10: 1 bit)")
      # "lato matteo:\n-rpm x100\n-marcia\n- velocità\n- engine temp \n- oil pressure (1 virgola mobile, /10)\n- battery voltage(1 virgola mobile, /10)."
      n163 = node-c288(i64 100 ("Period")) -> (w356:T2)  [unwired: 3 in]
      n164 = call-poly "VISA Configure Serial Port"("VISA resource name"=refnum<visa-resource-name> "ASRL1::INSTR", "Enable Termination\nChar (T)"=FALSE ("Enable Termination\nChar (T)"), "baud rate (9600)"=u32 4800, "data bits (8)"=u16 8, "parity (0:none)"=enum16{"None", "Odd", "Even", "Mark", "Space"}."None", "stop bits (10: 1 bit)"=w344) -> ("VISA resource name out"=w349:refnum<visa-resource-name>, "error out"=w350:errorcluster)  [unwired: 8 in]
      n165 = timed-loop {
        timing: w356 -> [_]
        timing-out: [_] -> w355
        tunnel: w350 -> [w379]
        tunnel: w349 -> [w378]
        tunnel: [w380] -> w347
        tunnel: [w377] -> w345
        stop <- w381 stop-if-true
        # "byte di start"
        n166 = node-c288() -> ()  [unwired: 1 in, 1 out]
        n167 = shared-variable "RT Single-Board RIO Target\\shared_var.lvlib\\Rpm"() -> (w373:u16)  [unwired: 1 in, 1 out]
        n168 = shared-variable "RT Single-Board RIO Target\\shared_var.lvlib\\Drive Speed"() -> (w368:dbl)  [unwired: 1 in, 1 out]
        n169 = shared-variable "RT Single-Board RIO Target\\shared_var.lvlib\\Battery Voltage"() -> (w358:sgl)  [unwired: 1 in, 1 out]
        n170 = shared-variable "RT Single-Board RIO Target\\shared_var.lvlib\\Engine Temp"() -> (w366:sgl)  [unwired: 1 in, 1 out]
        n171 = shared-variable "RT Single-Board RIO Target\\shared_var.lvlib\\Oil Pressure"() -> (w364:sgl)  [unwired: 1 in, 1 out]
        n172 = Divide(x=w373, y=u16 100) -> (x/y=w370:dbl)
        n173 = To Unsigned Byte Integer(number=w368) -> (unsigned 8bit integer=w367:u8)
        n174 = To Unsigned Byte Integer(number=w370) -> (unsigned 8bit integer=w369:u8)
        n175 = To Unsigned Byte Integer(number=w366) -> (unsigned 8bit integer=w365:u8)
        n176 = shared-variable "RT Single-Board RIO Target\\shared_var.lvlib\\Gear"() -> (w371:u8)  [unwired: 1 in, 1 out]
        n177 = Multiply(x=w358, y=sgl 10.0) -> (x*y=w359:sgl)
        n178 = Multiply(x=w364, y=sgl 10.0) -> (x*y=w363:sgl)
        n179 = To Unsigned Byte Integer(number=w359) -> (unsigned 8bit integer=w357:u8)
        n180 = To Unsigned Byte Integer(number=w363) -> (unsigned 8bit integer=w362:u8)
        n181 = local read "stop"() -> (w381:bool)
        n182 = Build Array(u8 204 ("element"), w369, w371, w367, w365, w362, w357) -> (w375:u8[])
        n183 = Byte Array To String(unsigned byte array=w375) -> (string=w376:string)
        n184 = node-c288() -> ()  [unwired: 1 in, 1 out]
        n185 = VISA Write(VISA resource name=w378, write buffer=w376, error in (no error)=w379) -> (VISA resource name out=w380:refnum<visa-resource-name>, error out=w377:errorcluster)  [unwired: 1 out]
      }
      n186 = node-c288(w355) -> ()  [unwired: 1 out]
      n187 = VISA Close(VISA resource name=w347, error in (no error)=w345) -> (error out=→"Error rs-232 display":errorcluster)
    }
    frame Disabled {
    }
  }
  n188 = node-c288() -> (w2:T2)  [unwired: 4 in]
  n189 = timed-loop {
    timing: w2 -> [_]
    timing-out: [_] -> w1
    stop <- FALSE stop-if-true
    n190 = node-c288() -> ()  [unwired: 1 in, 1 out]
    n191 = call <vilib>:"RT Get CPU Loads.vi"() -> ("CPU loads"=→"CPU loads":T1[])  [unwired: 10 in, 1 out]
    n192 = node-c288() -> ()  [unwired: 1 in, 1 out]
  }
  n193 = node-c288(w1) -> ()  [unwired: 1 out]
